vi "Write TestStatus.vi"(10 "TestStatus":T1 {"demandedProfileSteps" min=1; "demandedCycles" min=1; "activeProfileStep" min=1; "activeCycle" min=1}, 11 "Logger in":refnum<class "TestDataLog.lvclass">) -> (3 "Logger out":refnum<class "TestDataLog.lvclass">)   [LabVIEW 2015, in "TestDataLog.lvclass"]
uses:
  TestDataLog.lvclass
  Typedefs/TestStatus.ctl
  TestDataLog.lvclass/TestDataLog.ctl
  Typedefs/M1M3SSSTypedefs.lvlib
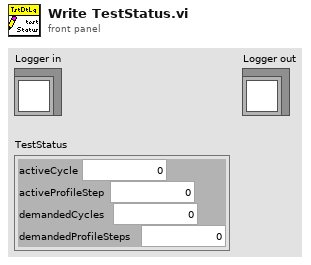
[diagram p1: front panel]
types:
  T1 = typedef "M1M3SSSTypedefs.lvlib/TestStatus.ctl" = cluster{"activeCycle":u32, "activeProfileStep":u32, "demandedCycles":u32, "demandedProfileSteps":u32}
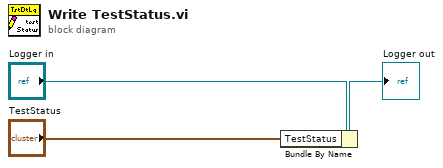
[diagram p0: block diagram]
diagram:
  n1 = Bundle By Name(cluster="Logger in", "TestStatus"="TestStatus") -> (→"Logger out":refnum<class "TestDataLog.lvclass">)
